vi "New.vi"(8 "error in (no error)":errorcluster, 11 "reference in":refnum<class "Switch_Manager.lvclass">) -> (0 "error out":errorcluster, 3 "reference out":refnum<class "Switch_Manager.lvclass">)   [LabVIEW 2022 SP3, in "Switch_Manager.lvlib" / "Switch_Manager.lvclass"]
uses:
  Switch_Manager.lvclass
  ObjectAttributes.ctl
  Components/SwitchBase.lvlibp/SwitchBase.lvclass
  Config.ctl
  SwitchMap.ctl
  Switch_Manager.lvclass/Switch_Manager.ctl
panel:
  in  "Data":T1
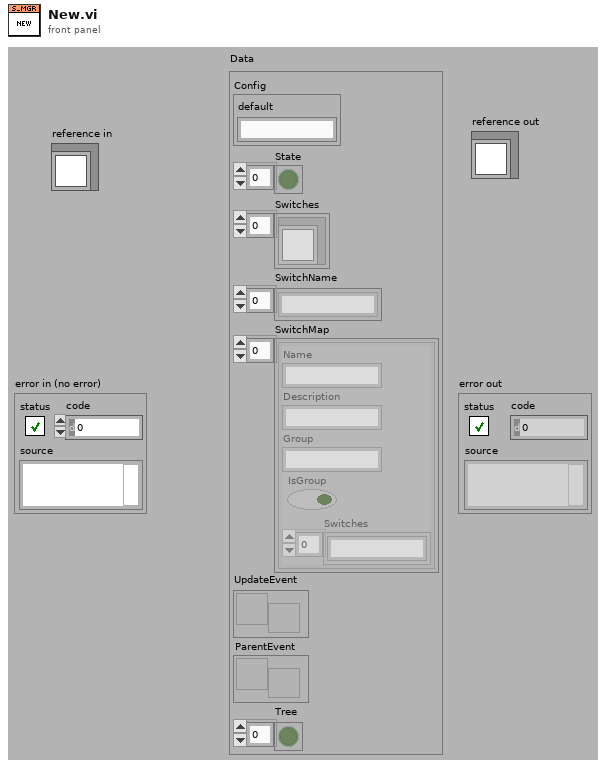
[diagram p1: front panel]
types:
  T1 = typedef "Switch_Manager.lvlib/Switch_Manager.lvclass/ObjectAttributes.ctl" = cluster{"Config":T2, "State":bool[], "Switches":refnum<class "SwitchBase.lvclass">[], "SwitchName":string[], "SwitchMap":T3[], "UpdateEvent":refnum<user-event>, "ParentEvent":refnum<user-event>, "Tree":bool[]}
  T2 = typedef "Switch_Manager.lvlib/Switch_Manager.lvclass/Config.ctl" = cluster{"default":string}
  T3 = typedef "Switch_Manager.lvlib/Switch_Manager.lvclass/SwitchMap.ctl" = cluster{"Name":string, "Description":string, "Group":string, "IsGroup":bool, "Switches":string[]}
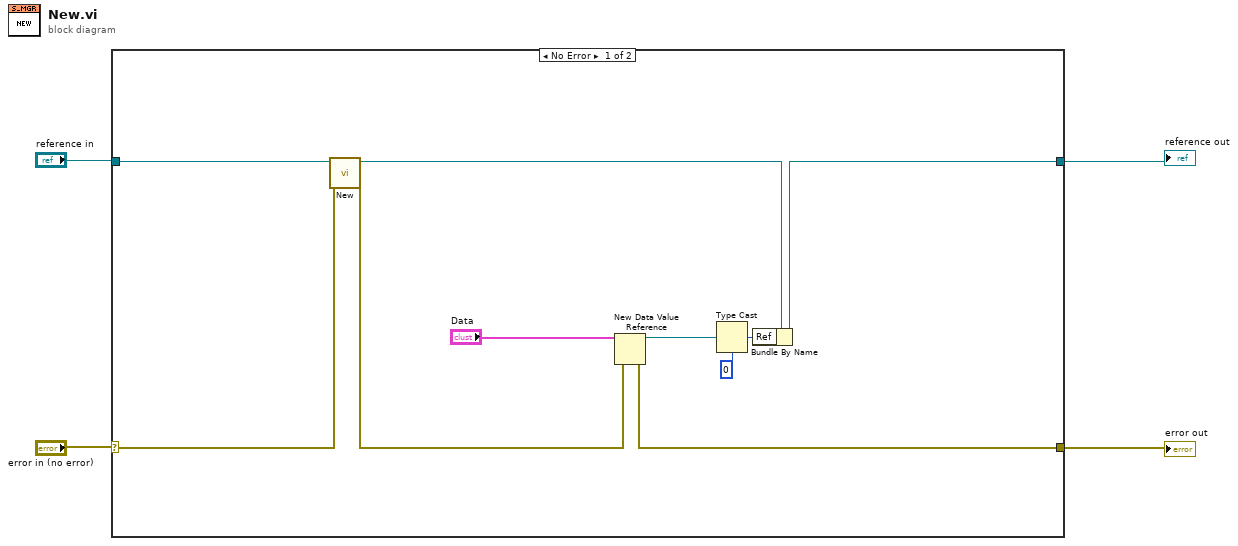
[diagram p0: block diagram]
diagram:
  n1 = case shown="No Error" "error in (no error)" {
    selector: "error in (no error)" -> [w7 w16]
    tunnel: [w5 w16] -> w2
    tunnel: "reference in" -> [w14 w15]
    tunnel: [w13 w15] -> w1
    frame No Error {
      n2 = call-parent "New.vi"("error in (no error)"=w7, "reference in"=w14) -> ("error out"=w6:errorcluster, "reference out"=w12:refnum<class "Switch_Manager.lvclass">)  [unwired: 8 in]
      n3 = New Data Value Reference(data value="Data", error in=w6) -> (data value reference=w10:refnum<data-value>, error out=w5:errorcluster)
      n4 = Type Cast(type=u32 0 ("DataRef"), x=w10) -> (*(type *) &x=w9:u32)
      n5 = Bundle By Name(cluster=w12, "Ref"=w9) -> (w13:refnum<class "Switch_Manager.lvclass">)
    }
    frame Error {
    }
  }
  "error out" <- w2
  "reference out" <- w1
